vi "Teleop.vi"(10 "Match Info":T1={"Autonomous Elapsed Seconds"=0.0, "TeleOp Elapsed Seconds"=0.0, "Disabled Elapsed Seconds"=0.0, "Visited Autonomous"=FALSE, "Visited TeleOp"=FALSE, "Visited Disabled"=FALSE, "Autonomous Settings"={"Autonomous Style"=enum."Independent", "VI Refnum"=refnum}}, 11 "Call Context":T2) -> ()   [LabVIEW 2017]
doc: "This VI is called for each TeleOp packet received from the DS where the robot is not disabled. It is often used to read from the joysticks and update I/O or to update setpoints for timed control loops. It should complete and return within 20 milliseconds or it may miss DS packets."
uses:
  <vilib>/Rock Robotics/WPI/DriverStation/WPI_DriverStationDerivedRobotMode.ctl
  <vilib>/Rock Robotics/WPI/DriverStation/WPI_DriverStationMatch Info.ctl
  <vilib>/Rock Robotics/Network Tables/NT Read Boolean.vi
  <vilib>/Rock Robotics/Network Tables/NT Read Number.vi
  <vilib>/Rock Robotics/WPI/Utilities/WPI_GetSetVariantRefNum.vi
  <vilib>/Rock Robotics/Network Tables/NT Write Boolean Array.vi
  <vilib>/Rock Robotics/Network Tables/NT Write Numeric Array.vi
  Robot Global Data.vi
panel:
  out "Sample Slider 0":dbl(slide) scale=0.0..5.0
  out "Sample Boolean 1":bool
  out "Sample Boolean 0":bool
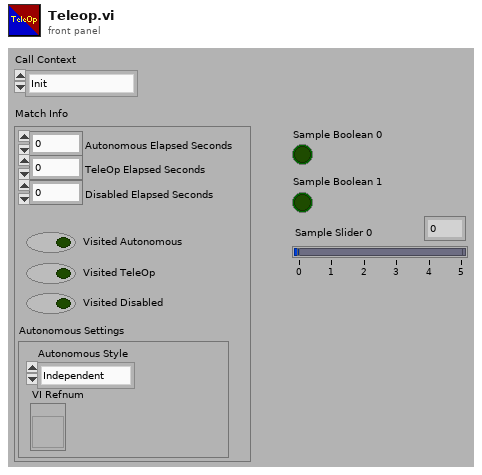
[diagram p1: front panel]
types:
  T1 = typedef "WPI_DriverStationMatch Info.ctl" = cluster{"Autonomous Elapsed Seconds":dbl, "TeleOp Elapsed Seconds":dbl, "Disabled Elapsed Seconds":dbl, "Visited Autonomous":bool, "Visited TeleOp":bool, "Visited Disabled":bool, "Autonomous Settings":cluster{"Autonomous Style":enum16{"Iterative", "Independent"}, "VI Refnum":refnum<vi>}}
  T2 = typedef "WPI_DriverStationDerivedRobotMode.ctl" = enum16{"Init", "Execute", "Stop"}
  T3 = typedef "WPI_JoystickDevRef.ctl" = cluster{"Device":T4}
  T4 = typedef "WPI_JoystickDeviceEnum.ctl" = enum16{"USB 0", "USB 1", "USB 2", "USB 3", "USB 4", "USB 5"}
  T5 = typedef "Control 1.ctl" = enum16{"SingleJoystick", "DoubleJoystick", "GameController"}
  T6 = cluster{"Buttons[0]":bool, "Buttons[1]":bool, "Buttons[2]":bool, "Buttons[3]":bool, "Buttons[4]":bool, "Buttons[5]":bool, "Buttons[6]":bool, "Buttons[7]":bool, "Buttons[8]":bool}
  T7 = cluster{"Axes[0]":dbl, "Axes[1]":dbl, "Axes[2]":dbl, "Axes[3]":dbl, "Axes[4]":dbl, "Axes[5]":dbl, "Axes[6]":dbl, "Axes[7]":dbl, "Axes[8]":dbl}
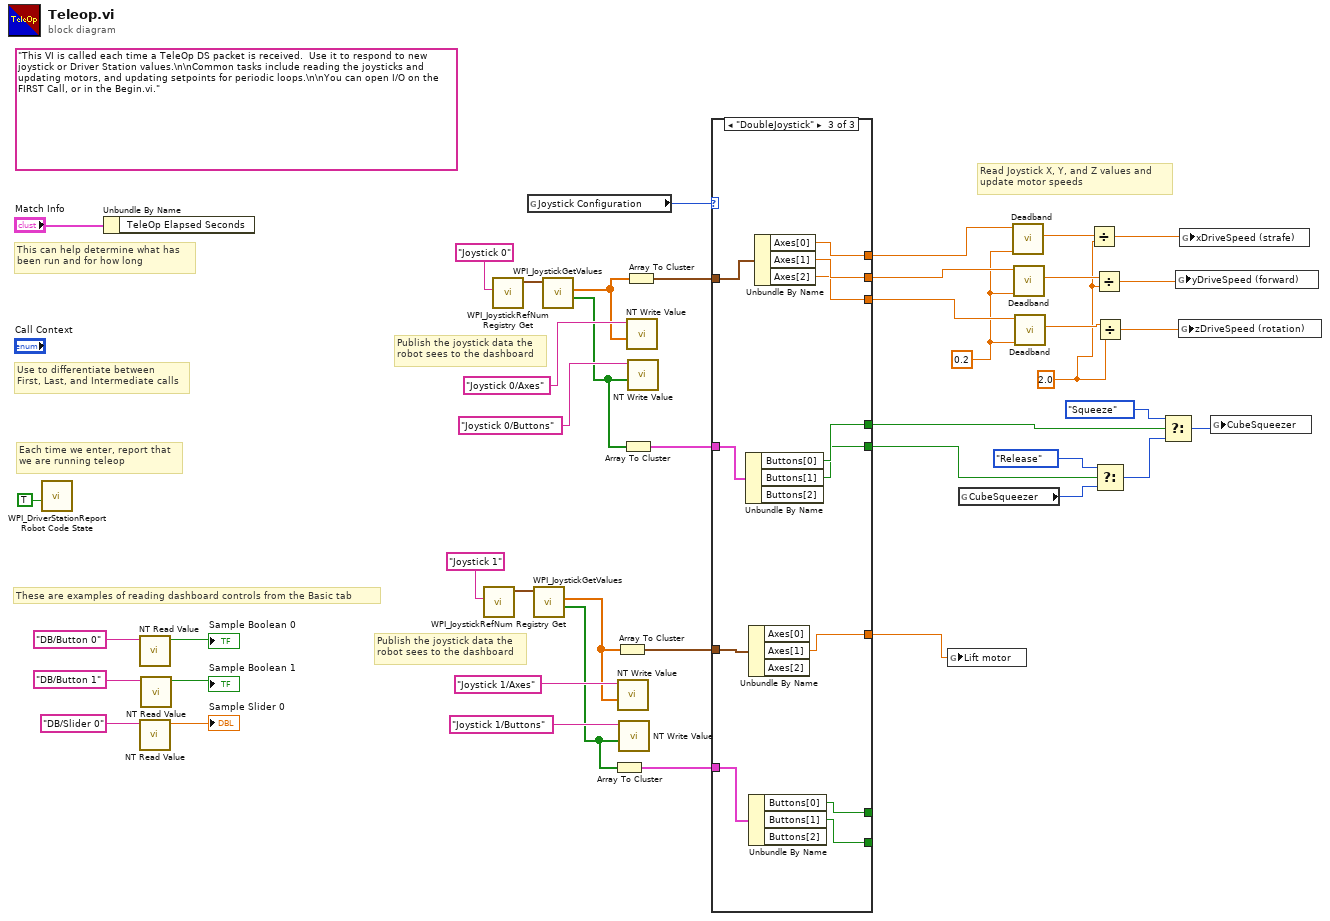
[diagram p0: block diagram]
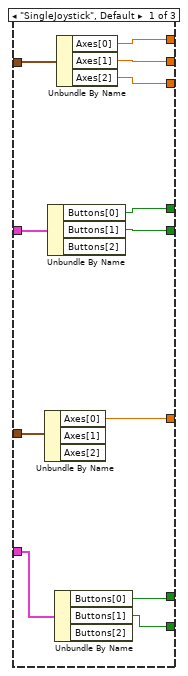
[diagram p2: hidden frame]
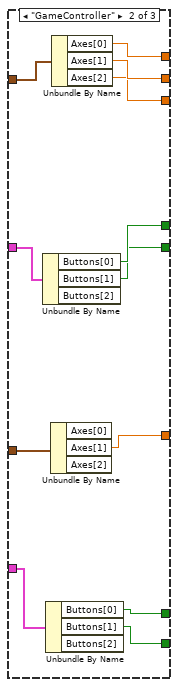
[diagram p3: hidden frame]
diagram:
  w5 = 2.0
  w23 = 0.2 ("guardband value")
  (unwired) "This VI is called each time a TeleOp DS packet is received.  Use it to respond to new joystick or Driver Station values.\n\nCommon tasks include reading the joysticks and updating motors, and updating setpoints for periodic loops.\n\nYou can open I/O on the FIRST Call, or in the Begin.vi."
  # "Publish the joystick data the\nrobot sees to the dashboard"
  # "Publish the joystick data the\nrobot sees to the dashboard"
  # "Read Joystick X, Y, and Z values and \nupdate motor speeds"
  # "These are examples of reading dashboard controls from the Basic tab"
  # "Each time we enter, report that\nwe are running teleop"
  # "Use to differentiate between\nFirst, Last, and Intermediate calls"
  # "This can help determine what has\nbeen run and for how long"
  n1 = call <vilib>:"WPI_DriverStationReport Robot Code State.vi"("TeleOp"=TRUE ("Autonomous")) -> ()  [unwired: 10 in, 1 out]
  n2 = Unbundle By Name("Match Info") -> ()  [unwired: 1 out]
  n3 = call-poly <vilib>:"NT Read Value.vi"("Name"="DB/Button 0" ("refnum name")) -> ("Boolean"=→"Sample Boolean 0":bool)  [unwired: 9 in, 1 out]
  n4 = call-poly <vilib>:"NT Read Value.vi"("Name"="DB/Slider 0" ("refnum name")) -> ("Numeric"=→"Sample Slider 0":dbl)  [unwired: 9 in, 1 out]
  n5 = call-poly <vilib>:"NT Read Value.vi"("Name"="DB/Button 1" ("refnum name")) -> ("Boolean"=→"Sample Boolean 1":bool)  [unwired: 9 in, 1 out]
  n6 = call <vilib>:"WPI_JoystickRefNum Registry Get.vi"("refnum name"="Joystick 1") -> ("JoystickDevRef"=w16:T3)  [unwired: 1 in, 9 out]
  n7 = call <vilib>:"WPI_JoystickRefNum Registry Get.vi"("refnum name"="Joystick 0") -> ("JoystickDevRef"=w35:T3)  [unwired: 1 in, 9 out]
  n8 = global read "Robot Global Data.vi" "Joystick Configuration"() -> (w9:T5)
  n9 = call <vilib>:"WPI_JoystickGetValues.vi"("JoystickDevRef"=w16) -> ("Buttons"=w11:bool[], "Axes"=w13:dbl[])  [unwired: 6 in, 3 out]
  n10 = call <vilib>:"WPI_JoystickGetValues.vi"("JoystickDevRef"=w35) -> ("Buttons"=w30:bool[], "Axes"=w32:dbl[])  [unwired: 6 in, 3 out]
  n11 = Array To Cluster(array=w11) -> (cluster=w10:T6)
  n12 = Array To Cluster(array=w13) -> (cluster=w12:T7)
  n13 = call-poly <vilib>:"NT Write Value.vi"("Numeric Array"=w13, "Name"="Joystick 1/Axes") -> ()  [unwired: 9 in, 1 out]
  n14 = call-poly <vilib>:"NT Write Value.vi"("Boolean Array"=w11, "Name"="Joystick 1/Buttons") -> ()  [unwired: 9 in, 1 out]
  n15 = Array To Cluster(array=w30) -> (cluster=w29:T6)
  n16 = Array To Cluster(array=w32) -> (cluster=w31:T7)
  n17 = call-poly <vilib>:"NT Write Value.vi"("Numeric Array"=w32, "Name"="Joystick 0/Axes") -> ()  [unwired: 9 in, 1 out]
  n18 = call-poly <vilib>:"NT Write Value.vi"("Boolean Array"=w30, "Name"="Joystick 0/Buttons") -> ()  [unwired: 9 in, 1 out]
  n19 = case shown="\"DoubleJoystick\"" w9 {
    tunnel: w31 -> [w56 w68 w80]
    tunnel: w29 -> [w55 w67 w79]
    tunnel: [w54 w66 w78] -> w28
    tunnel: [w53 w65 w77] -> w27
    tunnel: [w52 w64 w76] -> w26
    tunnel: [w51 w63 w75] -> w25
    tunnel: [w50 w62 w74] -> w24
    tunnel: w12 -> [w46 w58 w73]
    tunnel: w10 -> [w49 w61 w72]
    tunnel: [w48 w60 w71] -> _
    tunnel: [w47 w59 w70] -> _
    tunnel: [w45 w57 w69] -> w1
    frame "SingleJoystick", Default {
      n20 = Unbundle By Name(w46) -> ("Axes[0]"=w45:dbl)  [unwired: 2 out]
      n21 = Unbundle By Name(w55) -> ("Buttons[0]"=w51:bool, "Buttons[1]"=w50:bool)  [unwired: 1 out]
      n22 = Unbundle By Name(w49) -> ("Buttons[0]"=w48:bool, "Buttons[1]"=w47:bool)  [unwired: 1 out]
      n23 = Unbundle By Name(w56) -> ("Axes[0]"=w54:dbl, "Axes[1]"=w53:dbl, "Axes[2]"=w52:dbl)
    }
    frame "GameController" {
      n24 = Unbundle By Name(w67) -> ("Buttons[0]"=w63:bool, "Buttons[1]"=w62:bool)  [unwired: 1 out]
      n25 = Unbundle By Name(w61) -> ("Buttons[0]"=w60:bool, "Buttons[1]"=w59:bool)  [unwired: 1 out]
      n26 = Unbundle By Name(w58) -> ("Axes[1]"=w57:dbl)  [unwired: 2 out]
      n27 = Unbundle By Name(w68) -> ("Axes[0]"=w66:dbl, "Axes[1]"=w65:dbl, "Axes[2]"=w64:dbl)
    }
    frame "DoubleJoystick" {
      n28 = Unbundle By Name(w79) -> ("Buttons[0]"=w75:bool, "Buttons[1]"=w74:bool)  [unwired: 1 out]
      n29 = Unbundle By Name(w73) -> ("Axes[1]"=w69:dbl)  [unwired: 2 out]
      n30 = Unbundle By Name(w72) -> ("Buttons[0]"=w71:bool, "Buttons[1]"=w70:bool)  [unwired: 1 out]
      n31 = Unbundle By Name(w80) -> ("Axes[0]"=w78:dbl, "Axes[1]"=w77:dbl, "Axes[2]"=w76:dbl)
    }
  }
  n32 = global write "Robot Global Data.vi" "Lift motor"(w1) -> ()
  n33 = global read "Robot Global Data.vi" "CubeSqueezer"() -> (w22:enum16{"Squeeze", "Release"})
  n34 = call "Deadband.vi"("+- Bounds"=w23, "Raw Value"=w28) -> ("Filtered Value"=w8:dbl)  [unwired: 9 in]
  n35 = call "Deadband.vi"("+- Bounds"=w23, "Raw Value"=w27) -> ("Filtered Value"=w7:dbl)  [unwired: 9 in]
  n36 = call "Deadband.vi"("+- Bounds"=w23, "Raw Value"=w26) -> ("Filtered Value"=w6:dbl)  [unwired: 9 in]
  n37 = Divide(x=w8, y=w5) -> (x/y=w2:dbl)
  n38 = Divide(x=w7, y=w5) -> (x/y=w3:dbl)
  n39 = Divide(x=w6, y=w5) -> (x/y=w4:dbl)
  n40 = Select(t=enum16{"Squeeze", "Release"}."Release" ("CubeSqueezer"), s=w24, f=w22) -> (s? t:f=w18:enum16{"Squeeze", "Release"})
  n41 = Select(t=enum16{"Squeeze", "Release"}."Squeeze" ("CubeSqueezer"), s=w25, f=w18) -> (s? t:f=w19:enum16{"Squeeze", "Release"})
  n42 = global write "Robot Global Data.vi" "yDriveSpeed (forward)"(w3) -> ()
  n43 = global write "Robot Global Data.vi" "zDriveSpeed (rotation)"(w4) -> ()
  n44 = global write "Robot Global Data.vi" "xDriveSpeed (strafe)"(w2) -> ()
  n45 = global write "Robot Global Data.vi" "CubeSqueezer"(w19) -> ()
